vi "CI-recieveStatus.vi"(8 "error in (no error)":errorcluster, 10 "status":T1, 11 "common-interface in":refnum<class "CI-common_interface.lvclass">) -> (0 "error out":errorcluster, 3 "common-interface out":refnum<class "CI-common_interface.lvclass">)   [LabVIEW 2020, in "CI-common_interface.lvclass"]
uses:
  CI-common_interface.lvclass
  CI-status_clust.ctl
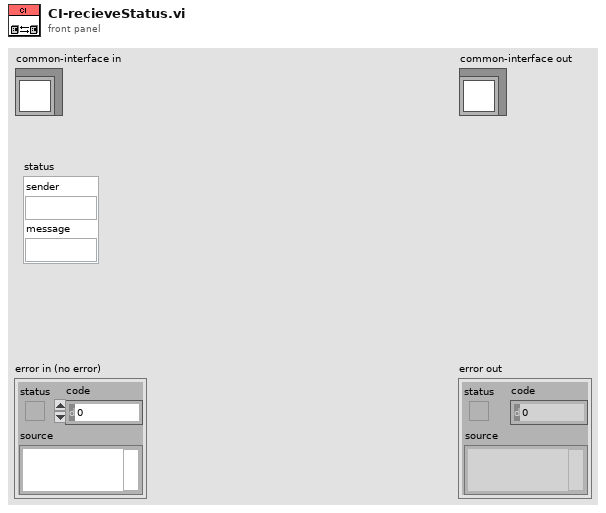
[diagram p1: front panel]
types:
  T1 = typedef "CI-common_interface.lvclass/CI-status_clust.ctl" = cluster{"sender":string, "message":string}
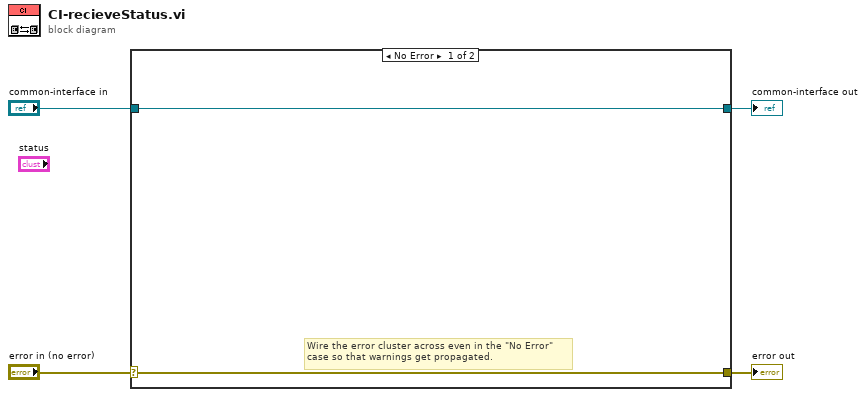
[diagram p0: block diagram]
diagram:
  n1 = case shown="No Error" "error in (no error)" {
    selector: "error in (no error)" -> [w5 w8]
    tunnel: [w5 w8] -> w3
    tunnel: [w6 w7] -> w1
    tunnel: "common-interface in" -> [w6 w7]
    frame No Error {
      # "Wire the error cluster across even in the \"No Error\"\ncase so that warnings get propagated."
    }
    frame Error {
    }
  }
  "error out" <- w3
  "common-interface out" <- w1
